vi "Byte array to hex string.vi"(11 "Array":u8[](array[numeric]) format="%x") -> (3 "String":string)   [LabVIEW 2020]
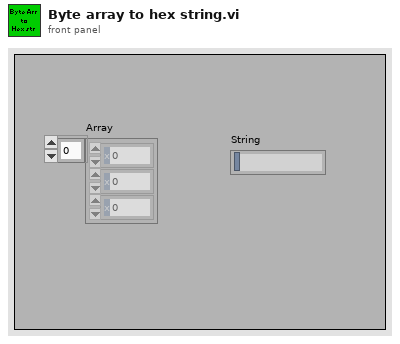
[diagram p1: front panel]
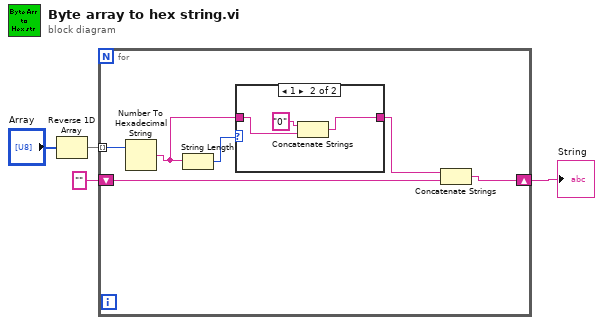
[diagram p0: block diagram]
diagram:
  n1 = Reverse 1D Array(array="Array") -> (reversed array=w1:u8[])
  n2 = for {
    shift-right: [w5] -> w4
    shift-left: "" -> [w10]
    tunnel: w1 -> [w9] mode=indexing
    n3 = Number To Hexadecimal String(2:w9) -> (0:w7:string)  [unwired: 1 in]
    n4 = String Length(string=w7) -> (length=w8:i32)
    n5 = case shown="1" w8 {
      tunnel: w7 -> [w11 w14]
      tunnel: [w11 w12] -> w6
      frame Default {
      }
      frame 1 {
        n6 = Concatenate Strings("0", w14) -> (w12:string)
      }
    }
    n7 = Concatenate Strings(w6, w10) -> (w5:string)
  }
  "String" <- w4
